vi "WiiMote Read Accelerometer.vi"(2 "error in":errorcluster, 3 "AccelState":refnum<k24>, 4 "WiimoteState":refnum<k24>, 5 "read raw values":bool) -> (0 "error out":errorcluster, 1 "Wiimote State":T1)   [LabVIEW 2015]
uses:
  C:/Users/gilled/Downloads/EmbeddedLab_v1.70_Courseware-Kobuki/EmbeddedLab_v1.70_Courseware/Courseware/src/LabVIEW/WiiMote/Dependencies/WiimoteLib.dll
  Dependencies/WiimoteLib.dll
  WiiMote State.ctl
panel:
  # "Accelerometers"
  # "Buttons"
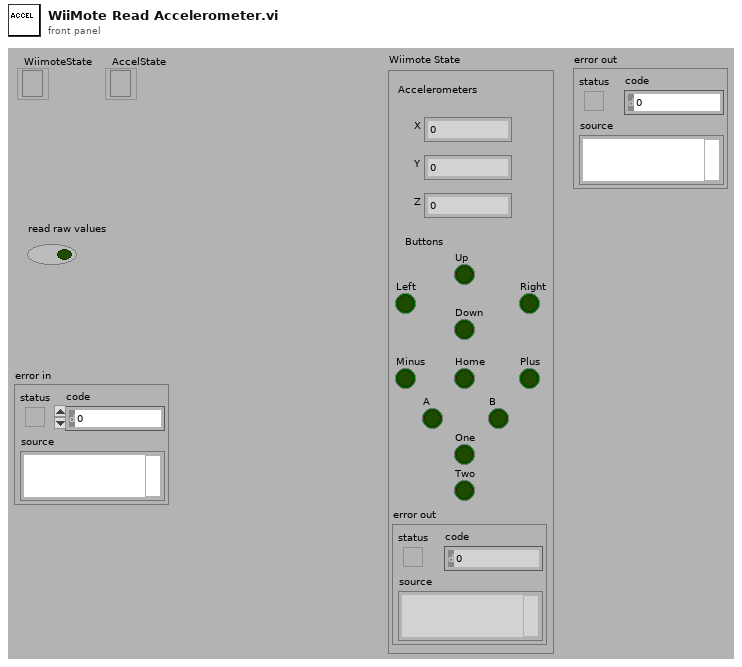
[diagram p1: front panel]
types:
  T1 = typedef "WiiMote State.ctl" = cluster{"X":sgl, "Y":sgl, "Z":sgl, "A":bool, "B":bool, "Down":bool, "Home":bool, "Left":bool, "Minus":bool, "One":bool, "Plus":bool, "Right":bool, "Two":bool, "Up":bool, "error out":errorcluster}
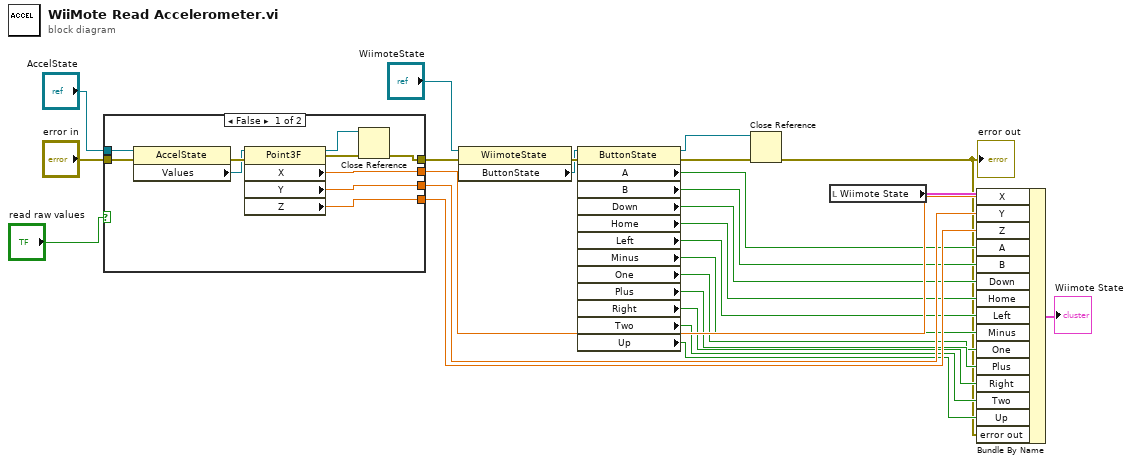
[diagram p0: block diagram]
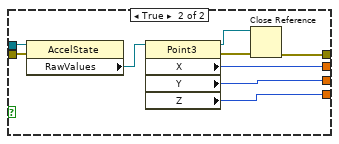
[diagram p2: hidden frame]
diagram:
  n1 = case shown="False" "read raw values" {
    tunnel: [w27 w37] -> w26
    tunnel: "error in" -> [w36 w44]
    tunnel: [w34 w40] -> w19
    tunnel: [w33 w41] -> w18
    tunnel: [w32 w42] -> w17
    tunnel: "AccelState" -> [w31 w45]
    frame False {
      n2 = property class="AccelState"(reference=w31, error in=w36) -> (error out=w35:errorcluster, "Values"=w30:refnum<k24>)  [unwired: 1 out]
      n3 = property class="Point3F"(reference=w30, error in=w35) -> (reference out=w29:refnum<k24>, error out=w28:errorcluster, "X"=w32:sgl, "Y"=w33:sgl, "Z"=w34:sgl)
      n4 = Close Reference(reference=w29, error in (no error)=w28) -> (error out=w27:errorcluster)
    }
    frame True {
      n5 = property class="AccelState"(reference=w45, error in=w44) -> ("RawValues"=w43:refnum<k24>)  [unwired: 2 out]
      n6 = property class="Point3"(reference=w43) -> (reference out=w38:refnum<k24>, error out=w39:errorcluster, "X"=w42:i32, "Y"=w41:i32, "Z"=w40:i32)  [unwired: 1 in]
      n7 = Close Reference(reference=w38, error in (no error)=w39) -> (error out=w37:errorcluster)
    }
  }
  n8 = property class="WiimoteState"(reference="WiimoteState", error in=w26) -> (error out=w22:errorcluster, "ButtonState"=w21:refnum<k24>)  [unwired: 1 out]
  n9 = property class="ButtonState"(reference=w21, error in=w22) -> (reference out=w23:refnum<k24>, error out=w24:errorcluster, "A"=w5:bool, "B"=w6:bool, "Down"=w7:bool, "Home"=w8:bool, "Left"=w9:bool, "Minus"=w10:bool, "One"=w11:bool, "Plus"=w12:bool, "Right"=w13:bool, "Two"=w14:bool, "Up"=w15:bool)
  n10 = Close Reference(reference=w23, error in (no error)=w24) -> (error out=w2:errorcluster)
  "error out" <- w2
  n11 = local read "Wiimote State"() -> (w3:T1)
  n12 = Bundle By Name(cluster=w3, "X"=w17, "Y"=w18, "Z"=w19, "A"=w5, "B"=w6, "Down"=w7, "Home"=w8, "Left"=w9, "Minus"=w10, "One"=w11, "Plus"=w12, "Right"=w13, "Two"=w14, "Up"=w15, "error out"=w2) -> (→"Wiimote State":T1)
